vi "create_state_queue.vi"(8 "error in (no error)":errorcluster) -> (0 "error out":errorcluster, 3 "Queue out":refnum<queue>)   [LabVIEW 2015]
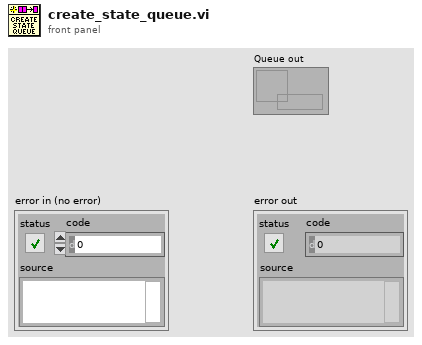
[diagram p1: front panel]
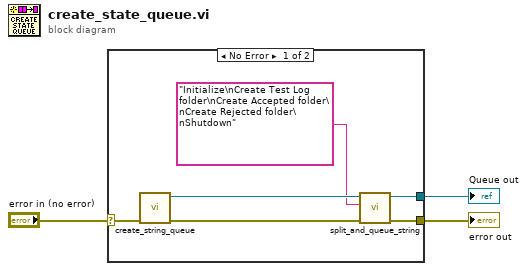
[diagram p0: block diagram]
diagram:
  n1 = case shown="No Error" "error in (no error)" {
    selector: "error in (no error)" -> [w4 w10]
    tunnel: [w6 _] -> w3
    tunnel: [w5 w10] -> w2
    frame No Error {
      n2 = call "create_string_queue.vi"("error in (no error)"=w4) -> ("error out"=w8:errorcluster, "Queue out"=w9:refnum<queue>)  [unwired: 9 in]
      n3 = call "split_and_queue_string.vi"("error in (no error)"=w8, "list state:argument"="Initialize\nCreate Test Log folder\nCreate Accepted folder\nCreate Rejected folder\nShutdown", "Queue in"=w9) -> ("error out"=w5:errorcluster, "Queue out"=w6:refnum<queue>)  [unwired: 7 in]
    }
    frame Error {
    }
  }
  "error out" <- w2
  "Queue out" <- w3
